vi "Sequencer Do.vi"(8 "error in (no error)":errorcluster, 10 "Sequencer in":refnum<class "Sequencer.lvclass">, 11 "Interrupt Sequencer Msg":refnum<class "Interrupt Sequncer Msg.lvclass">) -> (0 "error out":errorcluster, 2 "Sequencer out":refnum<class "Sequencer.lvclass">)   [LabVIEW 2020, in "Sequencer.lvlib" / "Interrupt Sequncer Msg.lvclass"]
doc: "The action the Sequencer Msg performs in the Sequencers Recieve Message method.\n\nThis implementation sends an interrupt on the Interrupt Notifier in the Sequencer Core."
uses:
  Interrupt Sequncer Msg.lvclass
  Sequencer/Sequencer.lvclass
  Sequencer/Sequencer.lvclass/Sequencer.ctl
  Sequencer Core/Sequencer Core.lvclass/Sequencer Core.ctl
  PPL/HDH.Data.Generic.lvlibp/Synchronization/Notifier/Send.vi
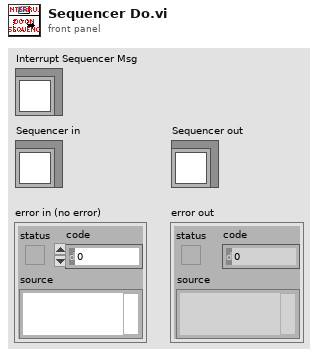
[diagram p1: front panel]
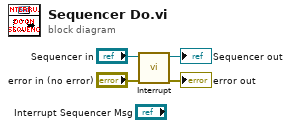
[diagram p0: block diagram]
diagram:
  n1 = call "Interrupt.vi"("error in (no error)"="error in (no error)", "Sequencer in"="Sequencer in") -> ("error out"=→"error out":errorcluster, "Sequencer out"=→"Sequencer out":refnum<class "Sequencer.lvclass">)  [unwired: 8 in]
